vi "APLUS Single Phase System.vi"(0 "Modbus Master in":refnum<class "Modbus Master.lvclass">, 1 "Reset WattHours":bool, 2 "Power Input":T2 {"Voltage (V):Element 1 Avg" format="%.3g"; "Voltage (V):Element 2 Avg" format="%.3g"; "Max Watt Hours" format="%.3g"; "Power Factor:Element 2" format="%.3g"; "Power Factor:Element 1" format="%.3g"; "Apparent Power (VA):Element 2" format="%.3g"; "Apparent Power (VA):Element 1" format="%.3g"; "Frequency (Hz):Element 1" format="%.3g"; "Time:Element 1" format="%.3g"; "Voltage Crest Factor:Element 2" format="%.3g"; "Voltage Crest Factor:Element 1" format="%.3g"; "Voltage Harmonic (%):Element 2" format="%.3g"; "Voltage Harmonic (%):Element 1" format="%.3g"; "Current Crest Factor:Element 2" format="%.3g"; "Current Crest Factor:Element 1" format="%.3g"; "Voltage (V):Element 1" format="%.3g"; "Voltage (V):Element 2" format="%.3g"; "Watt Hours (Wh):Sigma" format="%.3f"; "Power (W):Sigma" format="%.3g"; "Current (A):Element 2" format="%.3e"; "Current (A):Element 1" format="%.3e"}, 5 "error in (no error)":errorcluster) -> (8 "Holding Registers":u16[](array[numeric]), 12 "Power":sgl, 14 "Modbus Master out":refnum<class "Modbus Master.lvclass">, 16 "PowerData":T2 {"Voltage (V):Element 1 Avg" format="%.3g"; "Voltage (V):Element 2 Avg" format="%.3g"; "Max Watt Hours" format="%.3g"; "Power Factor:Element 2" format="%.3g"; "Power Factor:Element 1" format="%.3g"; "Apparent Power (VA):Element 2" format="%.3g"; "Apparent Power (VA):Element 1" format="%.3g"; "Frequency (Hz):Element 1" format="%.3g"; "Time:Element 1" format="%.3g"; "Voltage Crest Factor:Element 2" format="%.3g"; "Voltage Crest Factor:Element 1" format="%.3g"; "Voltage Harmonic (%):Element 2" format="%.3g"; "Voltage Harmonic (%):Element 1" format="%.3g"; "Current Crest Factor:Element 2" format="%.3g"; "Current Crest Factor:Element 1" format="%.3g"; "Voltage (V):Element 1" format="%.3g"; "Voltage (V):Element 2" format="%.3g"; "Watt Hours (Wh):Sigma" format="%.3f"; "Power (W):Sigma" format="%.3g"; "Current (A):Element 2" format="%.3e"; "Current (A):Element 1" format="%.3e"}, 19 "error out":errorcluster)   [LabVIEW 2019]
uses:
  <vilib>/NI/Modbus Library/API/Master/Modbus Master.lvclass
  C:/Program Files (x86)/National Instruments/LabVIEW 2019/vi.lib/NI/Modbus Library/API/Modbus API.lvclass
  Trunk/Utility/Type Definitions/UTILITY Power Data.ctl
  Type Definitions/APLUS Commands.ctl
panel:
  in  "Vthd":T1=235 items=["L1 Voltage (V) -14"=99, "L1 Voltage (V) -4U"=101, "L2 Voltage (V) -4U"=103, "L1 RMS Current (Amps) -14"=115, "L1 RMS Current (Amps) -4U"=117, "L2 RMS Current (Amps) -4U"=119, "Frequency (Hz) -All"=157, "Sys Power (Watts)-14"=133, "L1 Power (Watts)-4U"=135, "L2 Power (Watts)-4U"=137, "L1 Power Factor-14"=159, "L1 Power Factor-4U"=161, "L2 Power Factor-4U"=163, "L1 Apparent Power (VA)-14"=149, "L1 Apparent Power (VA)-4U"=151, "L2 Apparent Power (VA)-4U"=153, "Voltage Total Harmonic Distortion (%)-All"=235, "Active Energy Incoming-14"=1579, "Unit Factor-14"=1627, "Remainder Active Energy Incoming-14"=5999, "System Type"=2199]
  in  "Apparent Power":T1=149 items=["L1 Voltage (V) -14"=99, "L1 Voltage (V) -4U"=101, "L2 Voltage (V) -4U"=103, "L1 RMS Current (Amps) -14"=115, "L1 RMS Current (Amps) -4U"=117, "L2 RMS Current (Amps) -4U"=119, "Frequency (Hz) -All"=157, "Sys Power (Watts)-14"=133, "L1 Power (Watts)-4U"=135, "L2 Power (Watts)-4U"=137, "L1 Power Factor-14"=159, "L1 Power Factor-4U"=161, "L2 Power Factor-4U"=163, "L1 Apparent Power (VA)-14"=149, "L1 Apparent Power (VA)-4U"=151, "L2 Apparent Power (VA)-4U"=153, "Voltage Total Harmonic Distortion (%)-All"=235, "Active Energy Incoming-14"=1579, "Unit Factor-14"=1627, "Remainder Active Energy Incoming-14"=5999, "System Type"=2199]
  in  "Power Factor":T1=159 items=["L1 Voltage (V) -14"=99, "L1 Voltage (V) -4U"=101, "L2 Voltage (V) -4U"=103, "L1 RMS Current (Amps) -14"=115, "L1 RMS Current (Amps) -4U"=117, "L2 RMS Current (Amps) -4U"=119, "Frequency (Hz) -All"=157, "Sys Power (Watts)-14"=133, "L1 Power (Watts)-4U"=135, "L2 Power (Watts)-4U"=137, "L1 Power Factor-14"=159, "L1 Power Factor-4U"=161, "L2 Power Factor-4U"=163, "L1 Apparent Power (VA)-14"=149, "L1 Apparent Power (VA)-4U"=151, "L2 Apparent Power (VA)-4U"=153, "Voltage Total Harmonic Distortion (%)-All"=235, "Active Energy Incoming-14"=1579, "Unit Factor-14"=1627, "Remainder Active Energy Incoming-14"=5999, "System Type"=2199]
  in  "Power":T1=133 items=["L1 Voltage (V) -14"=99, "L1 Voltage (V) -4U"=101, "L2 Voltage (V) -4U"=103, "L1 RMS Current (Amps) -14"=115, "L1 RMS Current (Amps) -4U"=117, "L2 RMS Current (Amps) -4U"=119, "Frequency (Hz) -All"=157, "Sys Power (Watts)-14"=133, "L1 Power (Watts)-4U"=135, "L2 Power (Watts)-4U"=137, "L1 Power Factor-14"=159, "L1 Power Factor-4U"=161, "L2 Power Factor-4U"=163, "L1 Apparent Power (VA)-14"=149, "L1 Apparent Power (VA)-4U"=151, "L2 Apparent Power (VA)-4U"=153, "Voltage Total Harmonic Distortion (%)-All"=235, "Active Energy Incoming-14"=1579, "Unit Factor-14"=1627, "Remainder Active Energy Incoming-14"=5999, "System Type"=2199]
  in  "Frequency":T1=157 items=["L1 Voltage (V) -14"=99, "L1 Voltage (V) -4U"=101, "L2 Voltage (V) -4U"=103, "L1 RMS Current (Amps) -14"=115, "L1 RMS Current (Amps) -4U"=117, "L2 RMS Current (Amps) -4U"=119, "Frequency (Hz) -All"=157, "Sys Power (Watts)-14"=133, "L1 Power (Watts)-4U"=135, "L2 Power (Watts)-4U"=137, "L1 Power Factor-14"=159, "L1 Power Factor-4U"=161, "L2 Power Factor-4U"=163, "L1 Apparent Power (VA)-14"=149, "L1 Apparent Power (VA)-4U"=151, "L2 Apparent Power (VA)-4U"=153, "Voltage Total Harmonic Distortion (%)-All"=235, "Active Energy Incoming-14"=1579, "Unit Factor-14"=1627, "Remainder Active Energy Incoming-14"=5999, "System Type"=2199]
  in  "Current":T1=115 items=["L1 Voltage (V) -14"=99, "L1 Voltage (V) -4U"=101, "L2 Voltage (V) -4U"=103, "L1 RMS Current (Amps) -14"=115, "L1 RMS Current (Amps) -4U"=117, "L2 RMS Current (Amps) -4U"=119, "Frequency (Hz) -All"=157, "Sys Power (Watts)-14"=133, "L1 Power (Watts)-4U"=135, "L2 Power (Watts)-4U"=137, "L1 Power Factor-14"=159, "L1 Power Factor-4U"=161, "L2 Power Factor-4U"=163, "L1 Apparent Power (VA)-14"=149, "L1 Apparent Power (VA)-4U"=151, "L2 Apparent Power (VA)-4U"=153, "Voltage Total Harmonic Distortion (%)-All"=235, "Active Energy Incoming-14"=1579, "Unit Factor-14"=1627, "Remainder Active Energy Incoming-14"=5999, "System Type"=2199]
  in  "Voltage":T1=99 items=["L1 Voltage (V) -14"=99, "L1 Voltage (V) -4U"=101, "L2 Voltage (V) -4U"=103, "L1 RMS Current (Amps) -14"=115, "L1 RMS Current (Amps) -4U"=117, "L2 RMS Current (Amps) -4U"=119, "Frequency (Hz) -All"=157, "Sys Power (Watts)-14"=133, "L1 Power (Watts)-4U"=135, "L2 Power (Watts)-4U"=137, "L1 Power Factor-14"=159, "L1 Power Factor-4U"=161, "L2 Power Factor-4U"=163, "L1 Apparent Power (VA)-14"=149, "L1 Apparent Power (VA)-4U"=151, "L2 Apparent Power (VA)-4U"=153, "Voltage Total Harmonic Distortion (%)-All"=235, "Active Energy Incoming-14"=1579, "Unit Factor-14"=1627, "Remainder Active Energy Incoming-14"=5999, "System Type"=2199]
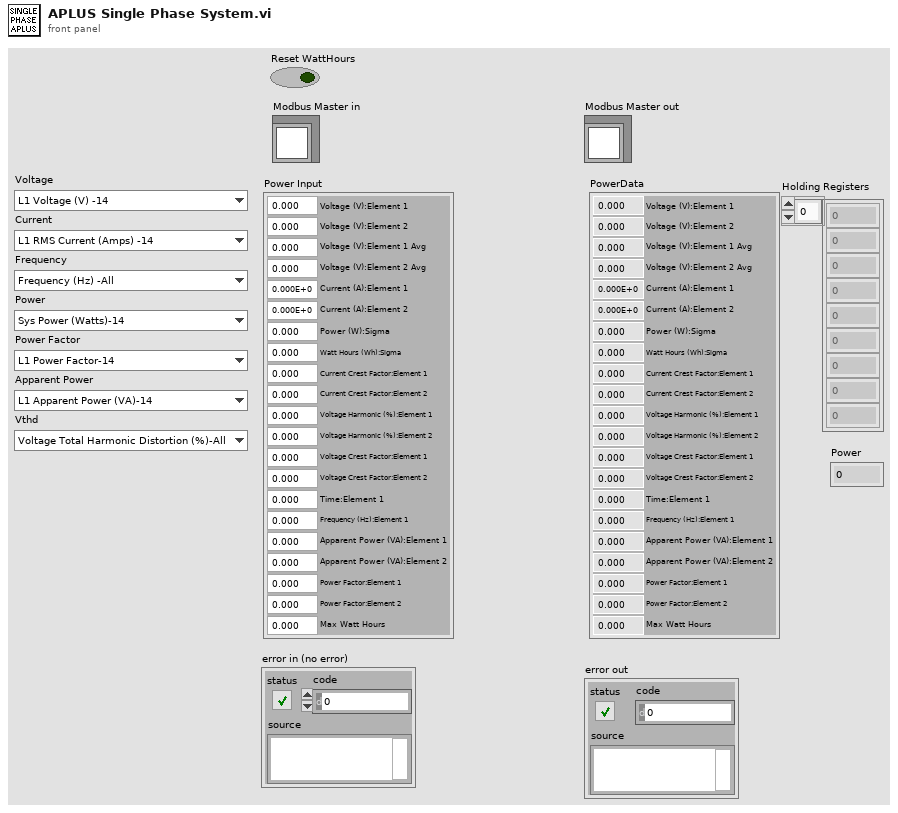
[diagram p1: front panel]
types:
  T1 = typedef "APLUS Commands.ctl" = u16
  T2 = typedef "UTILITY Power Data.ctl" = cluster{"Current (A):Element 1":dbl, "Current (A):Element 2":dbl, "Power (W):Sigma":dbl, "Watt Hours (Wh):Sigma":dbl, "Voltage (V):Element 2":dbl, "Voltage (V):Element 1":dbl, "Current Crest Factor:Element 1":dbl, "Current Crest Factor:Element 2":dbl, "Voltage Harmonic (%):Element 1":dbl, "Voltage Harmonic (%):Element 2":dbl, "Voltage Crest Factor:Element 1":dbl, "Voltage Crest Factor:Element 2":dbl, "Time:Element 1":dbl, "Frequency (Hz):Element 1":dbl, "Apparent Power (VA):Element 1":dbl, "Apparent Power (VA):Element 2":dbl, "Power Factor:Element 1":dbl, "Power Factor:Element 2":dbl, "Max Watt Hours":dbl, "Voltage (V):Element 2 Avg":dbl, "Voltage (V):Element 1 Avg":dbl}
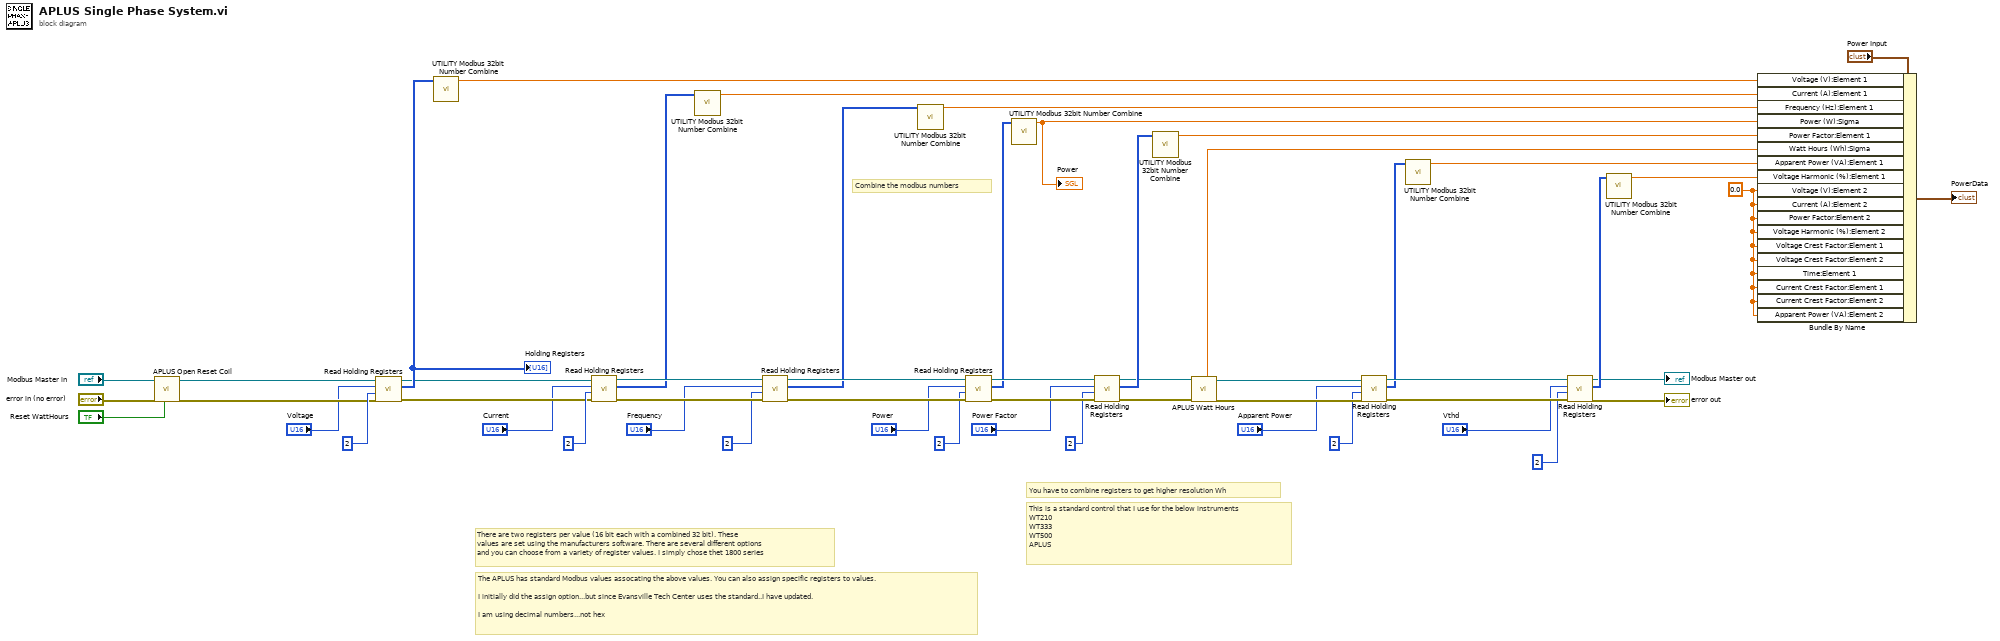
[diagram p0: block diagram]
diagram:
  w1 = 0.0 ("Urms:Element 2")
  # "The APLUS has standard Modbus values assocating the above values. You can also assign specific registers to values.\n\nI initially did the assign option...but since Evansville Tech Center uses the standard..I have updated.\n\nI am using decimal numbers...not hex"
  # "You have to combine registers to get higher resolution Wh"
  # "This is a standard control that I use for the below instruments\nWT210\nWT333\nWT500\nAPLUS"
  # "Combine the modbus numbers"
  # "There are two registers per value (16 bit each with a combined 32 bit). These \nvalues are set using the manufacturers software. There are several different options\nand you can choose from a variety of register values. I simply chose thet 1800 series"
  n1 = call "APLUS Open Reset Coil.vi"("Reset WattHours"="Reset WattHours", "error in (no error)"="error in (no error)", "Modbus Master in"="Modbus Master in") -> ("error out"=w24:errorcluster, "Modbus Master out"=w25:refnum<class "Modbus Master.lvclass">)  [unwired: 7 in]
  n2 = call-dynamic "Read Holding Registers.vi"("error in"=w24, "number of inputs"=u16 2 ("Quantity"), "starting address"="Voltage", "Modbus master in"=w25) -> ("error out"=w33:errorcluster, "register values"=w36:u16[], "Modbus master out"=w35:refnum<class "Modbus Master.lvclass">)  [unwired: 5 in]
  "Holding Registers" <- w36
  n3 = call "UTILITY Modbus 32bit Number Combine.vi"("Holding Registers"=w36) -> ("Data"=w9:sgl)  [unwired: 9 in, 1 out]
  n4 = call-dynamic "Read Holding Registers.vi"("error in"=w33, "number of inputs"=u16 2 ("Quantity"), "starting address"="Current", "Modbus master in"=w35) -> ("error out"=w45:errorcluster, "register values"=w26:u16[], "Modbus master out"=w49:refnum<class "Modbus Master.lvclass">)  [unwired: 5 in]
  n5 = call "UTILITY Modbus 32bit Number Combine.vi"("Holding Registers"=w26) -> ("Data"=w8:sgl)  [unwired: 9 in, 1 out]
  n6 = call-dynamic "Read Holding Registers.vi"("error in"=w45, "number of inputs"=u16 2 ("Quantity"), "starting address"="Frequency", "Modbus master in"=w49) -> ("error out"=w46:errorcluster, "register values"=w47:u16[], "Modbus master out"=w50:refnum<class "Modbus Master.lvclass">)  [unwired: 5 in]
  n7 = call "UTILITY Modbus 32bit Number Combine.vi"("Holding Registers"=w47) -> ("Data"=w7:sgl)  [unwired: 9 in, 1 out]
  n8 = call-dynamic "Read Holding Registers.vi"("error in"=w46, "number of inputs"=u16 2 ("Quantity"), "starting address"="Power", "Modbus master in"=w50) -> ("error out"=w51:errorcluster, "register values"=w48:u16[], "Modbus master out"=w53:refnum<class "Modbus Master.lvclass">)  [unwired: 5 in]
  n9 = call "UTILITY Modbus 32bit Number Combine.vi"("Holding Registers"=w48) -> ("Data"=w6:sgl)  [unwired: 9 in, 1 out]
  "Power" <- w6
  n10 = call-dynamic "Read Holding Registers.vi"("error in"=w51, "number of inputs"=u16 2 ("Quantity"), "starting address"="Power Factor", "Modbus master in"=w53) -> ("error out"=w44:errorcluster, "register values"=w52:u16[], "Modbus master out"=w43:refnum<class "Modbus Master.lvclass">)  [unwired: 5 in]
  n11 = call "UTILITY Modbus 32bit Number Combine.vi"("Holding Registers"=w52) -> ("Data"=w5:sgl)  [unwired: 9 in, 1 out]
  n12 = call "APLUS Watt Hours.vi"("error in (no error)"=w44, "Modbus instance in"=w43) -> ("error out"=w40:errorcluster, "Modbus instance out"=w38:refnum<class "Modbus Master.lvclass">, "Watt Hours"=w4:dbl)  [unwired: 7 in]
  n13 = call-dynamic "Read Holding Registers.vi"("error in"=w40, "number of inputs"=u16 2 ("Quantity"), "starting address"="Apparent Power", "Modbus master in"=w38) -> ("error out"=w39:errorcluster, "register values"=w41:u16[], "Modbus master out"=w42:refnum<class "Modbus Master.lvclass">)  [unwired: 5 in]
  n14 = call "UTILITY Modbus 32bit Number Combine.vi"("Holding Registers"=w41) -> ("Data"=w3:sgl)  [unwired: 9 in, 1 out]
  n15 = call-dynamic "Read Holding Registers.vi"("error in"=w39, "number of inputs"=u16 2 ("Quantity"), "starting address"="Vthd", "Modbus master in"=w42) -> ("error out"=→"error out":errorcluster, "register values"=w27:u16[], "Modbus master out"=→"Modbus Master out":refnum<class "Modbus Master.lvclass">)  [unwired: 5 in]
  n16 = call "UTILITY Modbus 32bit Number Combine.vi"("Holding Registers"=w27) -> ("Data"=w2:sgl)  [unwired: 9 in, 1 out]
  n17 = Bundle By Name(cluster="Power Input", "Voltage (V):Element 1"=w9, "Current (A):Element 1"=w8, "Frequency (Hz):Element 1"=w7, "Power (W):Sigma"=w6, "Power Factor:Element 1"=w5, "Watt Hours (Wh):Sigma"=w4, "Apparent Power (VA):Element 1"=w3, "Voltage Harmonic (%):Element 1"=w2, "Voltage (V):Element 2"=w1, "Current (A):Element 2"=w1, "Power Factor:Element 2"=w1, "Voltage Harmonic (%):Element 2"=w1, "Voltage Crest Factor:Element 1"=w1, "Voltage Crest Factor:Element 2"=w1, "Time:Element 1"=w1, "Current Crest Factor:Element 1"=w1, "Current Crest Factor:Element 2"=w1, "Apparent Power (VA):Element 2"=w1) -> (→"PowerData":T2)
